vi "split_averaging_filter.vi"(4 "Reset":bool, 8 "Parameters":T1, 10 "Noise":bool, 11 "Error":dbl[](array[numeric])) -> (0 "Order variance":dbl[](array[numeric]), 1 "Order mean":dbl[](array[numeric]), 2 "Variance":dbl[](array[numeric]), 3 "Prediction":dbl[](array[numeric]))   [LabVIEW 2014]
uses:
  averaging_filter_params.ctl
  <vilib>/Analysis/2dsp.llb/Real FFT.vi
  <vilib>/Analysis/2dsp.llb/Inverse Real FFT.vi
  <vilib>/Analysis/NI_AALPro.lvlib
panel:
  # "Signal minus previous prediction"
  # "Prediction for next data block, the same size as our input this time."
  # "If true, adaptation is supressed on this Error block"
  # "\"Order ...\" outputs are time domain models, with length \"Order\".   These are synchronous with the repeat period."
  # "Reset clears state to zeroes.  Filter must then settle to the steady-state output (multiple time constants)."
  # "Mean and variance of a repeating signal with known repeat period (order).  Input may be any length; mean and variance outputs are the same size as input.  This is like the averaging function on an oscilliscope.  As long as the time constant is much longer than the filter order, only signals that are synchronous with the order pass through into the mean.   In the frequency domain, we pass the order and harmonics of it.\n\nVariance is the filtered mean-squared difference between the input and the mean. This represents the expected variation at each position in the repeat period."
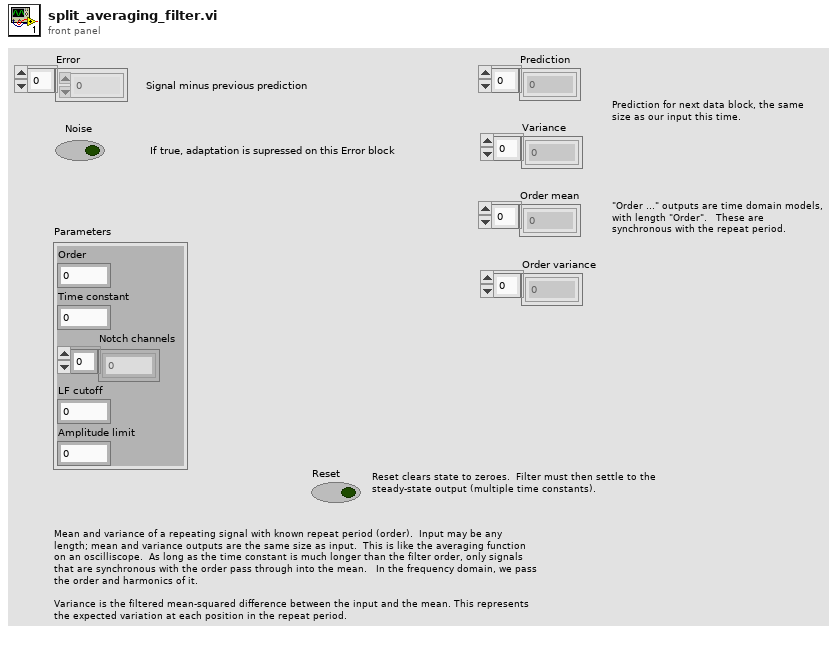
[diagram p1: front panel]
types:
  T1 = typedef "averaging_filter_params.ctl" = cluster{"Order":i32, "Time constant":dbl, "Notch channels":i32[], "LF cutoff":i32, "Amplitude limit":dbl}
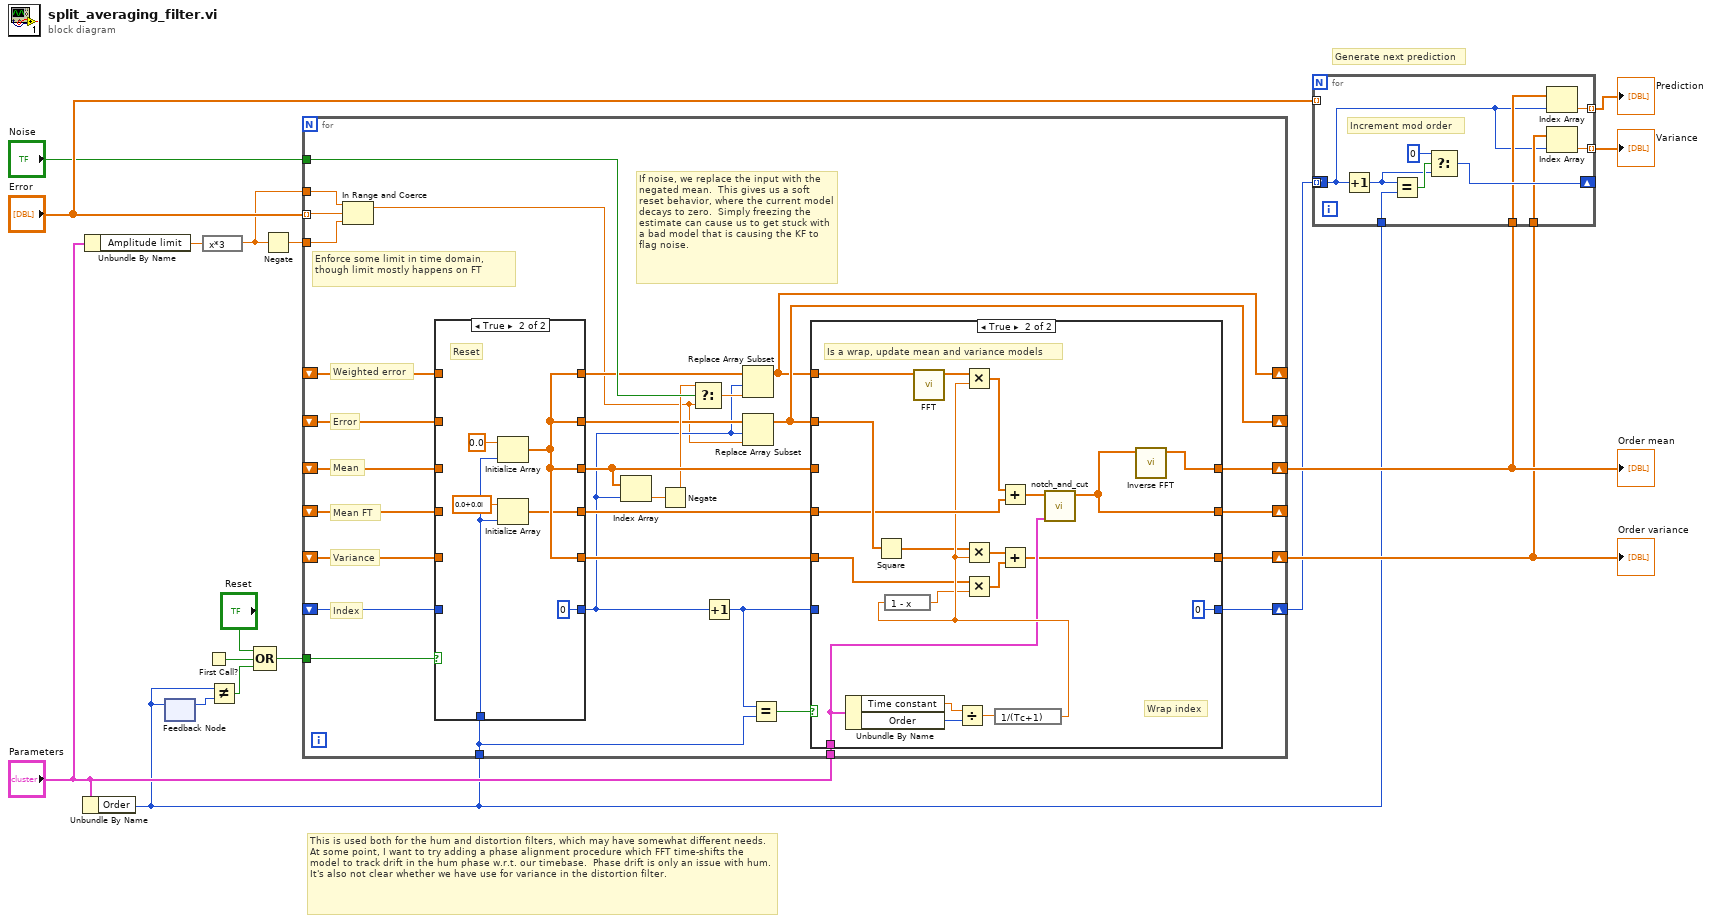
[diagram p0: block diagram]
diagram:
  # "Generate next prediction"
  # "This is used both for the hum and distortion filters, which may have somewhat different needs.  At some point, I want to try adding a phase alignment procedure which FFT time-shifts the model to track drift in the hum phase w.r.t. our timebase.  Phase drift is only an issue with hum.  It's also not clear whether we have use for variance in the distortion filter."
  n1 = Unbundle By Name("Parameters") -> ("Order"=w4:i32)
  n2 = Unbundle By Name("Parameters") -> ("Amplitude limit"=w7:dbl)
  n3 = feedback-in #1(w4) -> ()
  n4 = feedback #1() -> (w5:i32)  [unwired: 1 in]
  n5 = expression code="x*3"(w7) -> (w6:dbl)
  n6 = First Call?() -> (First Call?: T/F=w14:bool)
  n7 = Not Equal?(x=w4, y=w5) -> (x != y?=w3:bool)
  n8 = Compound Arithmetic op=OR("Reset", w14, w3) -> (w2:bool)
  n9 = Negate(x=w6) -> (-x=w8:dbl)
  n10 = for {
    tunnel: "Error" -> [w39] mode=indexing
    shift-right: [w48] -> w1
    shift-left: _ -> [w20]
    tunnel: w4 -> [w28]
    shift-right: [w41] -> _
    shift-left: _ -> [w31]
    shift-right: [w42] -> w11
    shift-left: _ -> [w29]
    shift-right: [w44] -> _
    shift-left: _ -> [w22]
    shift-right: [w43] -> _
    shift-left: _ -> [w24]
    shift-right: [w40] -> w10
    shift-left: _ -> [w32]
    tunnel: "Parameters" -> [w45]
    tunnel: "Noise" -> [w35]
    tunnel: w6 -> [w38]
    tunnel: w8 -> [w37]
    tunnel: w2 -> [w27]
    # "Index"
    # "Enforce some limit in time domain, though limit mostly happens on FT"
    # "Mean FT"
    # "Error"
    # "Weighted error"
    # "Mean"
    # "Variance"
    # "If noise, we replace the input with the negated mean.  This gives us a soft reset behavior, where the current model decays to zero.  Simply freezing the estimate can cause us to get stuck with a bad model that is causing the KF to flag noise."
    n11 = In Range and Coerce(upper limit=w38, x=w39, lower limit=w37) -> (coerced(x)=w18:dbl)  [unwired: 1 out]
    n12 = case shown="True" w27 {
      tunnel: w28 -> [_ w56]
      tunnel: w31 -> [w54 _]
      tunnel: [w54 w55] -> w30
      tunnel: [w53 w57] -> w26
      tunnel: w29 -> [w53 _]
      tunnel: [w49 0 ("Order")] -> w19
      tunnel: [w50 w57] -> w21
      tunnel: [w51 w57] -> w23
      tunnel: [w52 w57] -> w33
      tunnel: w32 -> [w52 _]
      tunnel: w24 -> [w51 _]
      tunnel: w22 -> [w50 _]
      tunnel: w20 -> [w49 _]
      frame False {
        # "Not reset"
      }
      frame True {
        # "Reset"
        n13 = Initialize Array(0.0 ("Decay"), w56) -> (w57:dbl[])
        n14 = Initialize Array(cdb 0.0+0.0i ("Decay"), w56) -> (w55:cdb[])
      }
    }
    n15 = Index Array(array=w26, index=w19) -> (element=w36:dbl)
    n16 = Negate(x=w36) -> (-x=w25:dbl)
    n17 = Select(t=w25, s=w35, f=w18) -> (s? t:f=w34:dbl)
    n18 = Increment(x=w19) -> (x+1=w47:i32)
    n19 = Replace Array Subset(array=w23, new element=w34, index=w19) -> (w43:dbl[])
    n20 = Replace Array Subset(array=w21, new element=w18, index=w19) -> (w44:dbl[])
    n21 = Equal?(x=w47, y=w28) -> (x = y?=w46:bool)
    n22 = case shown="True" w46 {
      tunnel: [w64 0] -> w48
      tunnel: w47 -> [w64 _]
      tunnel: w44 -> [_ w81]
      tunnel: w43 -> [_ w65]
      tunnel: w30 -> [w62 w79]
      tunnel: w45 -> [_ w69]
      tunnel: [w61 w76] -> w42
      tunnel: [w62 w75] -> w41
      tunnel: w33 -> [w63 w67]
      tunnel: [w63 w66] -> w40
      tunnel: w26 -> [w61 _]
      frame False {
        # "Not a wrap"
      }
      frame True {
        # "Wrap index"
        # "Is a wrap, update mean and variance models"
        n23 = Unbundle By Name(w69) -> ("Time constant"=w73:dbl, "Order"=w74:i32)
        n24 = Square(x=w81) -> (x^2=w68:dbl[])
        n25 = call-poly <vilib>:"FFT.vi"("X"=w65) -> ("FFT {X}"=w80:cdb[])  [unwired: 9 in, 1 out]
        n26 = Divide(x=w73, y=w74) -> (x/y=w72:dbl)
        n27 = expression code="1/(Tc+1)"(w72) -> (w71:dbl)
        n28 = expression code="1 - x"(w71) -> (w70:dbl)
        n29 = Multiply(x=w80, y=w71) -> (x*y=w78:cdb[])
        n30 = Multiply(x=w68, y=w71) -> (x*y=w82:dbl[])
        n31 = Multiply(x=w67, y=w70) -> (x*y=w83:dbl[])
        n32 = Add(x=w78, y=w79) -> (x+y=w77:cdb[])
        n33 = Add(x=w82, y=w83) -> (x+y=w66:dbl[])
        n34 = call "notch_and_cut.vi"("Parameters"=w69, "In"=w77) -> ("Out"=w75:cdb[])  [unwired: 9 in]
        n35 = call-poly <vilib>:"Inverse FFT.vi"("FFT {X}"=w75) -> ("X"=w76:dbl[])  [unwired: 9 in, 1 out]
      }
    }
  }
  "Order mean" <- w11
  "Order variance" <- w10
  n36 = for {
    shift-right: [w90] -> _
    shift-left: w1 -> [w85]
    tunnel: w4 -> [w93]
    tunnel: [w88] -> w15 mode=indexing
    tunnel: [w89] -> w16 mode=indexing
    tunnel: w10 -> [w87]
    tunnel: w11 -> [w86]
    tunnel: "Error" -> [_] mode=indexing
    tunnel: [w85] -> _ mode=indexing
    # "Increment mod order"
    n37 = Increment(x=w85) -> (x+1=w92:i32)
    n38 = Equal?(x=w92, y=w93) -> (x = y?=w94:bool)
    n39 = Select(t=0, s=w94, f=w92) -> (s? t:f=w90:i32)
    n40 = Index Array(array=w86, index=w85) -> (element=w88:dbl)
    n41 = Index Array(array=w87, index=w85) -> (element=w89:dbl)
  }
  "Prediction" <- w15
  "Variance" <- w16
